vi "Prime Factor.vi"(10 "n":i64) -> (3 "Prime Factors":i64[](array[numeric]))   [LabVIEW 2017, in "NI_AAL_MathFunc.lvlib"]
doc: "Computes the prime factorization of an integer."
uses:
  <vilib>/gmath/NI_AAL_MathFunc.lvlib
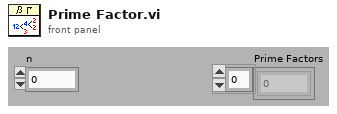
[diagram p1: front panel]
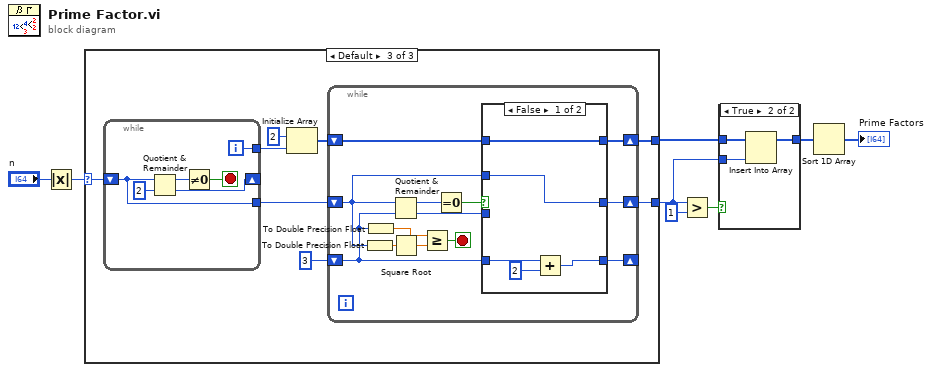
[diagram p0: block diagram]
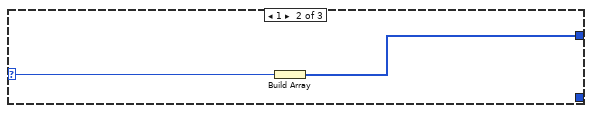
[diagram p4: hidden frame]
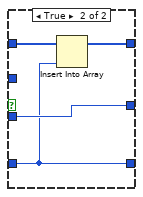
[diagram p5: hidden frame]
diagram:
  n1 = Absolute Value(x="n") -> (abs(x)=w6:i64)
  n2 = case shown="Default" w6 {
    selector: w6 -> [_ w10 w12]
    tunnel: [_ w9 w13] -> w5
    tunnel: [_ _ w11] -> w2
    frame 0 {
    }
    frame 1 {
      n3 = Build Array(w10) -> (w9:i64[])
    }
    frame Default {
      n4 = while {
        shift-right: [w42] -> _
        shift-left: w12 -> [w43]
        tunnel: [w43] -> w18
        tunnel: [w41] -> w17
        i -> [w41]
        stop <- w44 stop-if-true
        n5 = Quotient & Remainder(x=w43, y=i64 2) -> (x-y*floor(x/y)=w45:i64, floor(x/y)=w42:i64)
        n6 = Not Equal To 0?(x=w45) -> (x != 0?=w44:bool)
      }
      n7 = Initialize Array(i64 2 ("element"), w17) -> (w15:i64[])
      n8 = while {
        shift-right: [w26] -> w11
        shift-left: w18 -> [w21]
        shift-right: [w27] -> w13
        shift-left: w15 -> [w29]
        shift-right: [w25] -> _
        shift-left: i64 3 -> [w20]
        stop <- w23 stop-if-true
        n9 = To Double Precision Float(number=w21) -> (double precision float=w22:dbl)
        n10 = To Double Precision Float(number=w20) -> (double precision float=w19:dbl)
        n11 = Quotient & Remainder(x=w21, y=w20) -> (x-y*floor(x/y)=w31:i64, floor(x/y)=w28:i64)
        n12 = Square Root(x=w22) -> (sqrt(x)=w24:dbl)
        n13 = Greater Or Equal?(x=w19, y=w24) -> (x >= y?=w23:bool)
        n14 = Equal To 0?(x=w31) -> (x = 0?=w30:bool)
        n15 = case shown="False" w30 {
          tunnel: w29 -> [w36 w40]
          tunnel: w28 -> [_ w38]
          tunnel: w20 -> [w34 w37]
          tunnel: w21 -> [w35 _]
          tunnel: [w36 w39] -> w27
          tunnel: [w35 w38] -> w26
          tunnel: [w32 w37] -> w25
          frame False {
            n16 = Add(x=w34, y=i64 2) -> (x+y=w32:i64)
          }
          frame True {
            n17 = Insert Into Array(array=w40, new element=w37) -> (w39:i64[])  [unwired: 1 in]
          }
        }
      }
    }
  }
  n18 = Greater?(x=w2, y=i64 1) -> (0:w3:bool)
  n19 = case shown="True" w3 {
    tunnel: w5 -> [w47 w50]
    tunnel: [w47 w49] -> w1
    tunnel: w2 -> [_ w48]
    frame False {
    }
    frame True {
      n20 = Insert Into Array(array=w50, new element=w48) -> (w49:i64[])  [unwired: 1 in]
    }
  }
  n21 = Sort 1D Array(array=w1) -> (sorted array=→"Prime Factors":i64[])
